vi "fpga_Fund LP1 Filter.vi"(0 "input data":fxp<+/-,32,3>, 1 "reset":bool, 5 "#Ch":fxp<+,5,5>, 9 "input valid":bool) -> (4 "output data":fxp<+/-,32,4>, 10 "output valid":bool, 14 "ready for input":bool)   [LabVIEW 2012, in "NI_EP_Protection_FPGA.lvlib"]
doc: "----------------------\n\nThis filter is configured as follows:\n\n<b>Filter Configuration</b>\nType: Multirate - Decimation\nStructure: Polyphase FIR\nFactor: 8\n\n<b>Input Data Type</b>\nType: fixed-point <±,32,3> [-4.000000E+0,4.000000E+0]:1.862645E-9\n\n<b>Output Data Type</b>\nType: fixed-point <±,32,4> [-8.000000E+0,8.000000E+0]:3.725290E-9\nRounding mode: Truncate\nOverflow mode: Saturate\n\n<b>Implementation</b>\nNumber of channels: 16\nMaximum input sampling rate per channel @ 40MHz: 416.667kHz\nGain processing: On Host\nMethod: Multiply-Accumulate\nNumber of multiply pipeline stages: 1\nMultiply register in: False\nState memory: Block Memory\nCoefficient memory: ROM\n\n<b>Execution Mode</b>\nInside single-cycle Timed Loop\nThroughput: 6 cycles/sample\n\n<b>Estimated Resources</b>\nNumber of multiply-accumulate units: 1\nMultiply operation: I32.3 x I17.-2 => I48.4"
uses:
  <vilib>/addons/Electrical Power/Protection/NI_EP_Protection_FPGA.lvlib
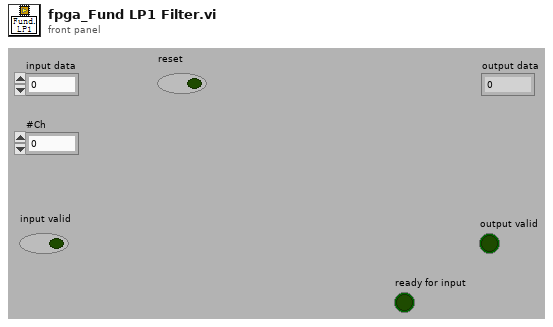
[diagram p1: front panel]
types:
  T1 = cluster{"WRSel":bool, "WREn":bool, "stateMemRDAddr":fxp<+,7,7>, "stateMemWRAddr":fxp<+,7,7>, "firstRun":bool}
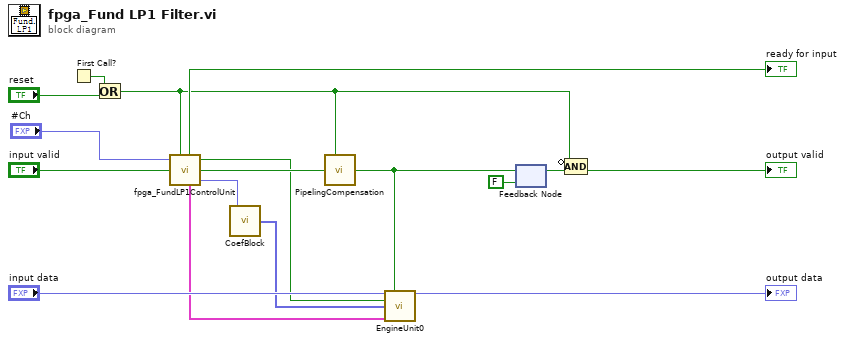
[diagram p0: block diagram]
diagram:
  n1 = First Call?() -> (First Call?: T/F=w12:bool)
  n2 = Or(x=w12, y="reset") -> (x .or. y?=w10:bool)
  n3 = call <vilib>:"fpga_FundLP1ControlUnit.vi"("#Ch"="#Ch", "reset"=w10, "input valid"="input valid") -> ("ready for input"=→"ready for input":bool, "procInputValid"=w7:bool, "output valid"=w14:bool, "opState"=w4:T1, "coefRDAddr"=w9:fxp<+,6,6>)  [unwired: 2 in]
  n4 = call "CoefBlock"("coefAddr"=w9) -> ("coefficients"=w5:fxp<+/-,17,-2>[])  [unwired: 8 in]
  n5 = call "PipelingCompensation"("reset"=w10, "data in"=w14) -> ("data out"=w6:bool)  [unwired: 7 in]
  n6 = call "EngineUnit0"("input data"="input data", "Output_Latch"=w6, "Input_Latch"=w7, "coefficients"=w5, "opState"=w4) -> ("output data"=→"output data":fxp<+/-,32,4>)  [unwired: 10 in]
  n7 = feedback-in #1(w6) -> ()
  n8 = feedback #1(FALSE ("procInputValid")) -> (w15:bool)
  n9 = Compound Arithmetic op=AND(invert w10, w15) -> (→"output valid":bool)
